vi "DeleteLastCrvs.vi"(8 "error in (no error)":errorcluster caption="entrée d'erreur (pas d'erreur)", 9 "defer update":bool, 10 "CurveNumber":i32, 11 "Interface en entrée":refnum<class "Interface.lvclass"> caption="DNL_LabVIEW Object in") -> (0 "error out":errorcluster caption="sortie d'erreur", 3 "Interface en sortie":refnum<class "Interface.lvclass"> caption="DNL_LabVIEW Object out")   [LabVIEW 2019, in "Interface.lvclass"]
uses:
  Interface.lvclass
  Interface.lvclass/Interface.ctl
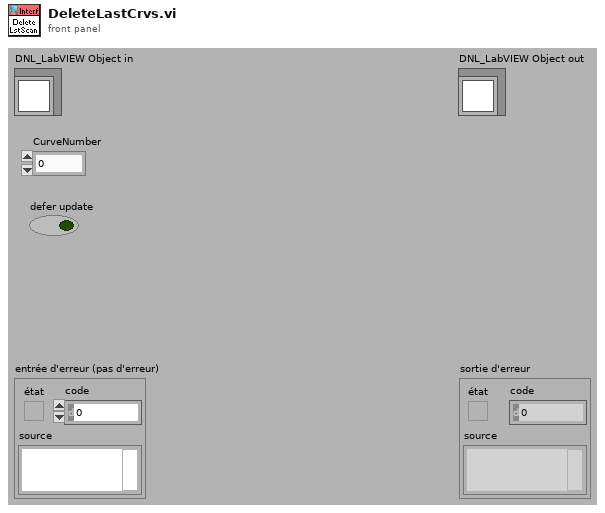
[diagram p1: front panel]
types:
  T1 = typedef "Interface.lvclass/CurveSetup.ctl" = cluster{"CurveName":string, "YParam":string, "XParam":string, "ZParam ":string, "GroupName":string, "LinWdth":u8, "PntCol":u32, "LinCol":u32, "LablFor":u8, "XScale":u32, "YScale":u32, "Interpol":u8, "DisplayName":string, "FillType":i16, "LineStyle":u8, "PntStyle":u8, "BarTyp":u8, "GraphIndex":i32, "Visible":bool, "XScaleName":string, "YScaleName":string, "XYGraph_Ref":refnum<vi>, "Data Only":bool, "DataQ Ref":refnum<queue>, "XParQ Ref":refnum<queue>, "XParamInd":i32, "ScanInd":i32, "File Path":path}
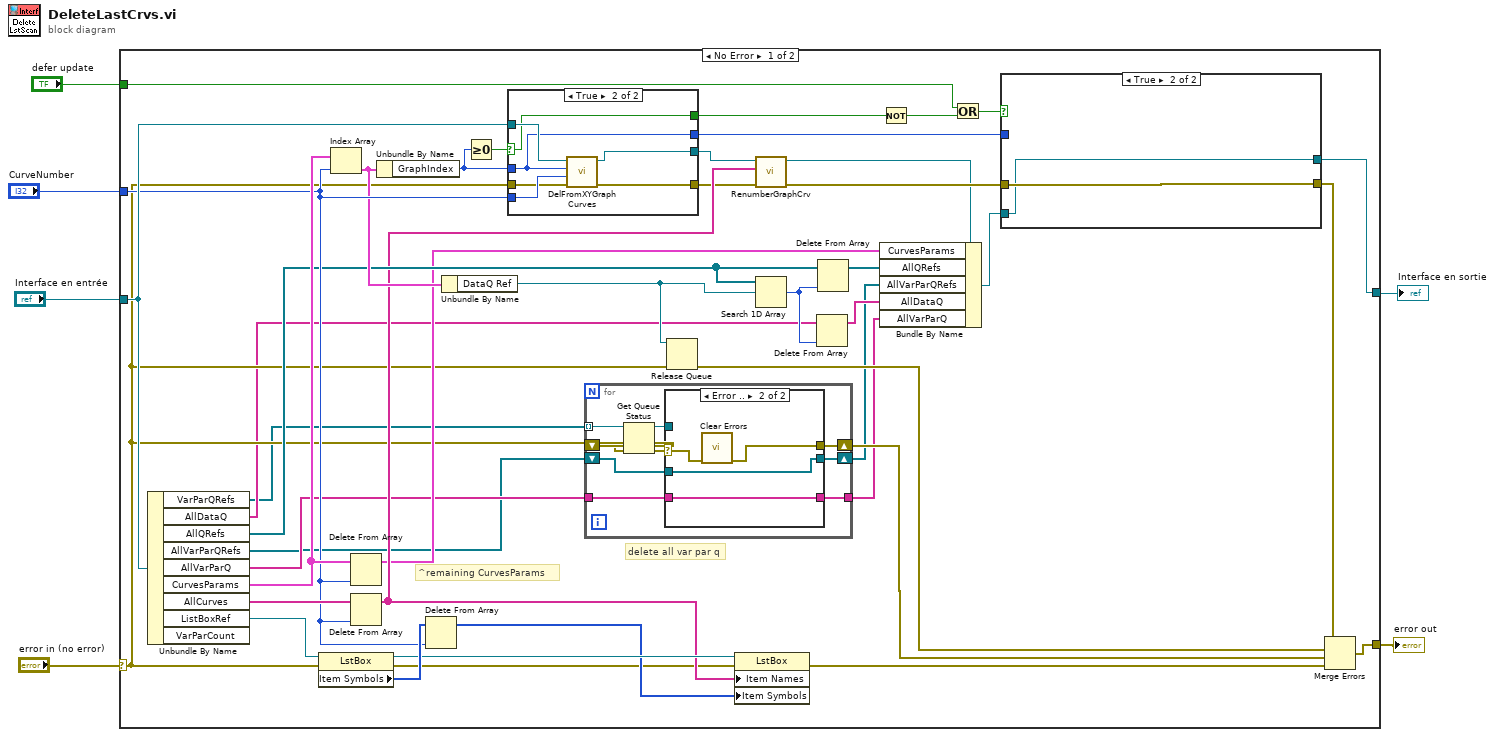
[diagram p0: block diagram]
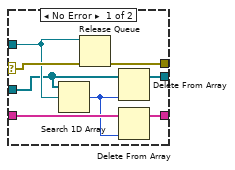
[diagram p2: hidden frame]
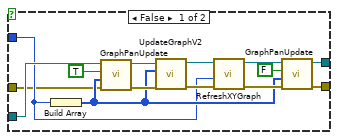
[diagram p3: hidden frame]
diagram:
  n1 = case shown="No Error" "error in (no error)" {
    selector: "error in (no error)" -> [w32 w98]
    tunnel: [w28 w98] -> w5
    tunnel: [w11 w97] -> w3
    tunnel: "Interface en entrée" -> [w47 w97]
    tunnel: "CurveNumber" -> [w42 _]
    tunnel: "defer update" -> [w7 _]
    frame No Error {
      # "delete all var par q"
      # "^remaining CurvesParams"
      n2 = Unbundle By Name(w47) -> ("VarParQRefs"=w16:refnum<queue>[], "AllDataQ"=w23:string[], "AllQRefs"=w38:refnum<queue>[], "AllVarParQRefs"=w12:refnum<queue>[], "AllVarParQ"=w15:string[], "CurvesParams"=w44:T1[], "AllCurves"=w45:string[], "ListBoxRef"=w46:refnum<vi>)  [unwired: 1 out]
      n3 = property class="LstBox"(reference=w46, error in=w32) -> (reference out=w41:refnum<vi>, error out=w33:errorcluster, "Item Symbols"=w43:i32[])
      n4 = Index Array(array=w44, index=w42) -> (element=w39:T1)
      n5 = Delete From Array(array=w44, index=w42) -> (array with subset deleted=w35:T1[])  [unwired: 1 in, 1 out]
      n6 = Delete From Array(array=w45, index=w42) -> (array with subset deleted=w36:string[])  [unwired: 1 in, 1 out]
      n7 = Unbundle By Name(w39) -> ("GraphIndex"=w48:i32)
      n8 = Delete From Array(array=w43, index=w42) -> (array with subset deleted=w40:i32[])  [unwired: 1 in, 1 out]
      n9 = Unbundle By Name(w39) -> ("DataQ Ref"=w37:refnum<queue>)
      n10 = Greater Or Equal To 0?(x=w48) -> (x >= 0?=w31:bool)
      n11 = case shown="True" w31 {
        selector: w31 -> [w88 w92]
        tunnel: w42 -> [_ w95]
        tunnel: w48 -> [w87 w93]
        tunnel: w47 -> [w86 w96]
        tunnel: w32 -> [w89 w94]
        tunnel: [w89 w90] -> w18
        tunnel: [w87 w93] -> w29
        tunnel: [w88 w92] -> w9
        tunnel: [w86 w91] -> w21
        frame False {
          # "curves was not graphed"
        }
        frame True {
          n12 = call "DelFromXYGraphCurves.vi"("error in (no error)"=w94, "CurvIndex"=w95, "GraphIndex"=w93, "Interface en entrée"=w96) -> ("error out"=w90:errorcluster, "Interface en sortie"=w91:refnum<class "Interface.lvclass">)  [unwired: 6 in]
        }
      }
      n13 = for {
        shift-right: [w57] -> w17
        shift-left: w32 -> [w53]
        tunnel: w16 -> [w54] mode=indexing
        tunnel: w15 -> [w56]
        tunnel: [w55] -> w14
        shift-right: [w49] -> w13
        shift-left: w12 -> [w50]
        n14 = Get Queue Status(queue=w54, error in (no error)=w53) -> (queue out=w52:refnum<queue>, error out=w51:errorcluster)  [unwired: 1 in, 6 out]
        n15 = case shown="Error .." w51 {
          selector: w51 -> [w62 w69]
          tunnel: [w65 w68] -> w57
          tunnel: w52 -> [w60 _]
          tunnel: w56 -> [w64 w67]
          tunnel: w50 -> [w59 w66]
          tunnel: [w63 w67] -> w55
          tunnel: [w61 w66] -> w49
          frame No Error {
            n16 = Search 1D Array(1D array=w59, element=w60) -> (index of element=w58:i32)  [unwired: 1 in]
            n17 = Release Queue(queue=w60, error in (no error)=w62) -> (error out=w65:errorcluster)  [unwired: 1 in, 2 out]
            n18 = Delete From Array(array=w59, index=w58) -> (array with subset deleted=w61:refnum<queue>[])  [unwired: 1 in, 1 out]
            n19 = Delete From Array(array=w64, index=w58) -> (array with subset deleted=w63:string[])  [unwired: 1 in, 1 out]
          }
          frame Error {
            n20 = call <vilib>:"Clear Errors.vi"("error in (no error)"=w69) -> ("error out"=w68:errorcluster)  [unwired: 5 in, 1 out]
          }
        }
      }
      n21 = Release Queue(queue=w37, error in (no error)=w32) -> (error out=w26:errorcluster)  [unwired: 1 in, 2 out]
      n22 = property class="LstBox"(reference=w41, error in=w33, "Item Names"=w36, "Item Symbols"=w40) -> (error out=w25:errorcluster)  [unwired: 1 out]
      n23 = call "RenumberGraphCrv.vi"("error in (no error)"=w18, "AllCurves"=w36, "Interface en entrée"=w21) -> ("error out"=w20:errorcluster, "Interface en sortie"=w19:refnum<class "Interface.lvclass">)  [unwired: 7 in]
      n24 = Search 1D Array(1D array=w38, element=w37) -> (index of element=w24:i32)  [unwired: 1 in]
      n25 = Delete From Array(array=w23, index=w24) -> (array with subset deleted=w22:string[])  [unwired: 1 in, 1 out]
      n26 = Delete From Array(array=w38, index=w24) -> (array with subset deleted=w34:refnum<queue>[])  [unwired: 1 in, 1 out]
      n27 = Bundle By Name(cluster=w19, "CurvesParams"=w35, "AllQRefs"=w34, "AllVarParQRefs"=w13, "AllDataQ"=w22, "AllVarParQ"=w14) -> (w30:refnum<class "Interface.lvclass">)
      n28 = Not(x=w9) -> (.not. x?=w8:bool)
      n29 = Or(x=w7, y=w8) -> (x .or. y?=w10:bool)
      n30 = case shown="True" w10 {
        tunnel: w30 -> [w74 w84]
        tunnel: w29 -> [w73 _]
        tunnel: w20 -> [w72 w85]
        tunnel: [w71 w85] -> w27
        tunnel: [w70 w84] -> w11
        frame False {
          n31 = Build Array(w73) -> (w78:i32[])
          n32 = call "GraphPanUpdate.vi"("error in (no error)"=w72, "GraphInd"=w78, "DeferUpdate"=TRUE, "Interface en entrée"=w74) -> ("error out"=w83:errorcluster, "Interface en sortie"=w82:refnum<class "Interface.lvclass">)  [unwired: 6 in]
          n33 = call "UpdateGraphV2.vi"("error in (no error)"=w83, "GraphIndexArr"=w78, "Interface en entrée"=w82) -> ("error out"=w77:errorcluster, "Interface en sortie"=w80:refnum<class "Interface.lvclass">)  [unwired: 7 in]
          n34 = call "RefreshXYGraph.vi"("error in (no error)"=w77, "Graph Index"=w73, "Interface en entrée"=w80) -> ("error out"=w79:errorcluster, "Interface en sortie"=w81:refnum<class "Interface.lvclass">)  [unwired: 6 in, 1 out]
          n35 = call "GraphPanUpdate.vi"("error in (no error)"=w79, "GraphInd"=w78, "DeferUpdate"=FALSE, "Interface en entrée"=w81) -> ("error out"=w71:errorcluster, "Interface en sortie"=w70:refnum<class "Interface.lvclass">)  [unwired: 6 in]
        }
        frame True {
        }
      }
      n36 = Merge Errors(w27, w26, w17, w25) -> (w28:errorcluster)
    }
    frame Error {
    }
  }
  "error out" <- w5
  "Interface en sortie" <- w3
